vi "1.3.1-Serial Read.vi"(0 "Rx FPGA I/O":refnum<k21>="Rx", 1 "Read FIFO":refnum<k21>="Read FIFO", 7 "baud rate (9600)":u32=9600, 9 "data bits (8)":i32=8 min=5 max=8 step=1, 11 "parity (0:none)":enum16{"None", "Odd", "Even", "Mark", "Space"}(ring), 12 "stop bits (10: 1 bit)":u16(ring)=10 items=["1.0"=10, "1.5"=15, "2.0"=20], 13 "Invert Polarity?":bool) -> ()   [LabVIEW 2010]
uses:
  <vilib>/eio/EIONode/EIONode.xnode
  <vilib>/rvi/eio/nirviEIOImplementation/nirviEIOImplementation.xnode
  <vilib>/rvi/eio/common/nirviEmuClasses.ctl
  <vilib>/rvi/DataTransferAndStorage/Container/XNode/niFpgaContainer.xnode
  <vilib>/rvi/DataTransferAndStorage/Container/Common/niFpgaTransferTypeControl.ctl
  <vilib>/rvi/FIFO/Fifo_Types/niFpgaFifoControlLogicControl.ctl
  <vilib>/rvi/DataTransferAndStorage/Container/Common/niFpgaContainerMethod.ctl
  <vilib>/rvi/DataTransferAndStorage/Container/Common/niFpgaContainerMetaDataKey.ctl
  <vilib>/rvi/DataTransferAndStorage/FIFO/niFpgaPeerToPeerStreamState.ctl
  1.0-Hindbrain Global.vi
  <vilib>/rvi/eio/common/nirviEmuTemplateMethod_noerrors.vi
  Instance           1 27Saved   LV FPGA Serial Read .vi
  Instance           2 27Saved   LV FPGA Serial Read .vi
  <vilib>/rvi/DataTransferAndStorage/Container/Common/niFpgaContainerExecOnDevCompGetState.vi
  <vilib>/rvi/FIFO/Fifo_Resource/nirvififoEmulationSetSize.vi
  <vilib>/rvi/DataTransferAndStorage/Container/Common/niFpgaContainerGetUniqueNameForEmu.vi
  <vilib>/rvi/interface/RandomDataEmulation/nirviRandomDataFPGAFIFO.vi
  <vilib>/rvi/interface/RandomDataEmulation/niFpgaRandomDataHandleErrors.vi
  <vilib>/rvi/eio/common/nirviEmuReportErrorAndStop.vi
  Instance           3 27Saved   LV FPGA Serial Read .vi
  Instance           6 27Saved   LV FPGA Serial Read .vi
panel:
  out "Read: Transmission Error":bool
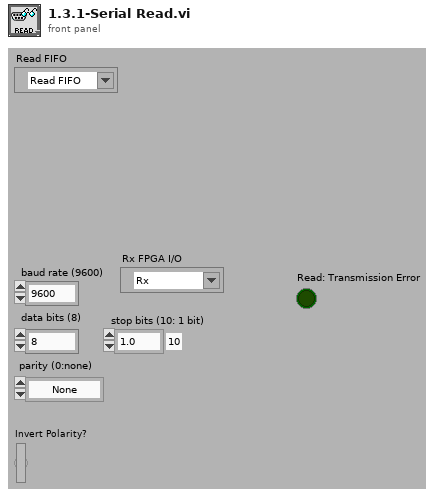
[diagram p1: front panel]
types:
  T1 = typedef "nirviEmuClasses.ctl" = enum16{"IO Read", "IO Write", "Method", "Property Read", "Property Write"}
  T2 = typedef "niFpgaFifoControlLogicControl.ctl" = enum16{"Slice Fabric", "Target Optimal", "Built-in"}
  T3 = typedef "niFpgaContainerMethod.ctl" = enum16{"<none>", "write", "read", "clear", "getNumberOfElementsToWrite", "getNumberOfElementsToRead", "enable", "disable", "flushAndDisable", "getStreamState", "readA", "readB", "dramWrite", "dramWriteWithByteEnables", "dramRequestData", "dramRetrieveData"}
  T4 = typedef "niFpgaTransferTypeControl.ctl" = enum16{"Target-Scoped", "Host to Target - DMA", "Target to Host - DMA", "Peer to Peer Reader", "Peer to Peer Writer", "Bidirectional"}
  T5 = typedef "niFpgaPeerToPeerStreamState.ctl" = enum16{"Unlinked", "Disabled", "Enabled", "Flushing"}
  T6 = typedef "niFpgaContainerMetaDataKey.ctl" = enum16{"FPGA FIFO", "FPGA Memory", "FPGA Register"}
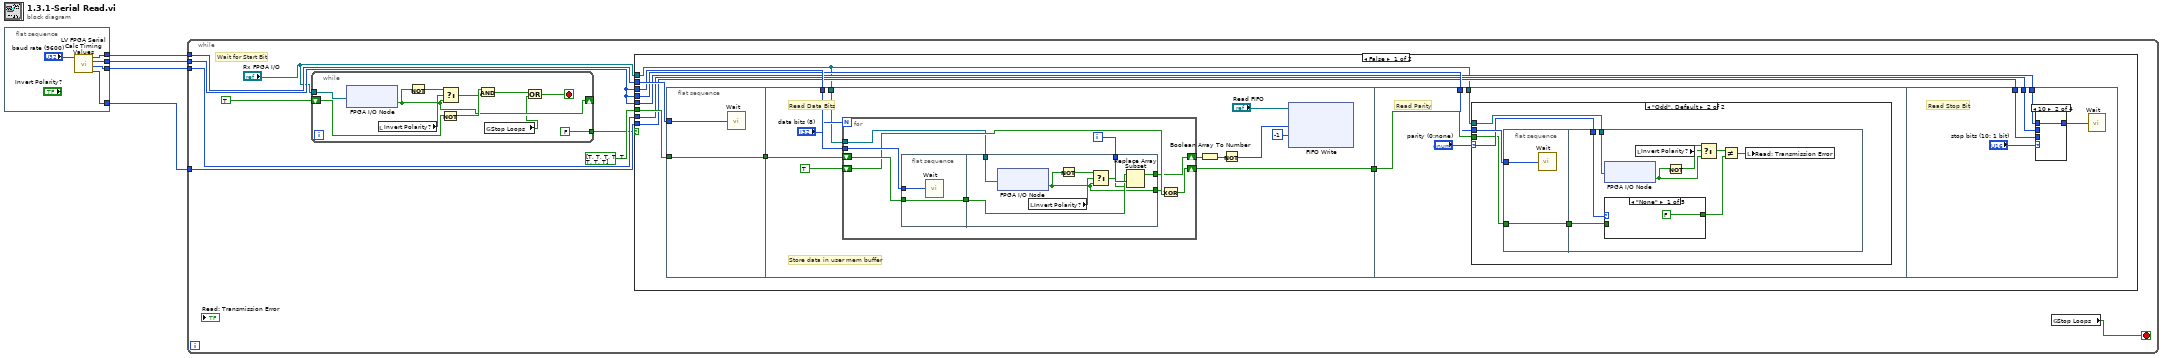
[diagram p0: block diagram]
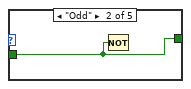
[diagram p3: hidden frame]
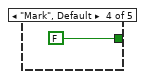
[diagram p5: hidden frame]
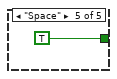
[diagram p6: hidden frame]
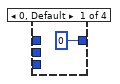
[diagram p7: hidden frame]
diagram:
  n1 = flat-sequence {
    tunnel: [w5] -> w3
    tunnel: [w8] -> w4
    tunnel: [w7] -> w2
    tunnel: [w6] -> w1
    frame #0 {
      n2 = call "LV FPGA Serial Calc Timing Values.vi"("baud rate (1000000)"="baud rate (9600)") -> ("Two Bit"=w6:u32, "One and Half Bit"=w7:u32, "One Bit"=w5:u32, "Half Bit"=w8:u32)  [unwired: 1 in, 2 out]
    }
  }
  n3 = while {
    tunnel: w1 -> [w17]
    tunnel: w2 -> [w16]
    tunnel: w3 -> [w15]
    tunnel: w4 -> [w14]
    stop <- w11 stop-if-true
    # "Wait for Start Bit"
    n4 = while {
      tunnel: [FALSE] -> w13
      shift-right: [w20] -> _
      shift-left: TRUE -> [w28]
      tunnel: "Rx FPGA I/O" -> [w24]
      stop <- w25 stop-if-true
      n5 = xnode "FPGA I/O Node"("FPGA I/O In"=w24) -> ("I/O Item"=w20:bool)  [unwired: 1 out]
      n6 = local read "Invert Polarity?"() -> (w22:bool)
      n7 = Not(x=w20) -> (.not. x?=w23:bool)
      n8 = Not(x=w28) -> (.not. x?=w27:bool)
      n9 = Select(t=w23, s=w22, f=w20) -> (s? t:f=w21:bool)
      n10 = And(x=w27, y=w21) -> (x .and. y?=w26:bool)
      n11 = global read "1.0-Hindbrain Global.vi" "Stop Loops"() -> (w19:bool)
      n12 = Or(x=w26, y=w19) -> (x .or. y?=w25:bool)
    }
    n13 = case shown="False" w13 {
      tunnel: bool[] [TRUE, TRUE, TRUE, TRUE, TRUE, TRUE, TRUE, TRUE] -> [w57 _]
      tunnel: w14 -> [w56 _]
      tunnel: w15 -> [w55 _]
      tunnel: w15 -> [w54 _]
      tunnel: w15 -> [w53 _]
      tunnel: w16 -> [w52 _]
      tunnel: w17 -> [w51 _]
      tunnel: "Rx FPGA I/O" -> [w49 _]
      frame False {
        n14 = flat-sequence {
          tunnel: [w60] -> w58
          tunnel: w57 -> [w60]
          tunnel: w56 -> [w59]
          tunnel: w58 -> [w71]
          tunnel: w55 -> [w70]
          tunnel: [w66] -> w50
          tunnel: w49 -> [w64]
          tunnel: w54 -> [w428]
          tunnel: w50 -> [w430]
          tunnel: w49 -> [w427]
          tunnel: w53 -> [w474]
          tunnel: w52 -> [w473]
          tunnel: w51 -> [w472]
          frame #0 {
            n15 = call "Wait"("Count(Ticks)"=w59) -> ()  [unwired: 1 out]
          }
          frame #1 {
            # "Store data in user mem buffer"
            # "Read Data Bits"
            n16 = for {
              N: "data bits (8)" -> [_]
              shift-right: [w391] -> w69
              shift-left: w71 -> [w397]
              tunnel: w70 -> [w395]
              shift-right: [w394] -> w66
              shift-left: TRUE -> [w393]
              tunnel: w64 -> [w389]
              i -> [w390]
              n17 = flat-sequence {
                tunnel: w397 -> [w399]
                tunnel: [w399] -> w396
                tunnel: w395 -> [w398]
                tunnel: w390 -> [w407]
                tunnel: w396 -> [w406]
                tunnel: [w405] -> w391
                tunnel: [w400] -> w392
                tunnel: w389 -> [w404]
                frame #0 {
                  n18 = call "Wait"("Count(Ticks)"=w398) -> ()  [unwired: 1 out]
                }
                frame #1 {
                  n19 = xnode "FPGA I/O Node"("FPGA I/O In"=w404) -> ("I/O Item"=w400:bool)  [unwired: 1 out]
                  n20 = local read "Invert Polarity?"() -> (w403:bool)
                  n21 = Not(x=w400) -> (.not. x?=w402:bool)
                  n22 = Select(t=w402, s=w403, f=w400) -> (s? t:f=w401:bool)
                  n23 = Replace Array Subset(array=w406, new element=w401, index=w407) -> (w405:bool[])
                }
              }
              n24 = Exclusive Or(1:w393, 2:w392) -> (0:w394:bool)
            }
            n25 = Boolean Array To Number(Boolean array=w69) -> (number=w68:u8)
            n26 = Not(x=w68) -> (.not. x?=w63:u8)
            n27 = xnode ("FIFO Write")("Element"=w63, "Timeout"=-1, "FIFO In"="Read FIFO") -> ()  [unwired: 2 out]
          }
          frame #2 {
            # "Read Parity"
            n28 = case shown="\"Odd\", Default" "parity (0:none)" {
              selector: "parity (0:none)" -> [_ w434]
              tunnel: w430 -> [_ w432]
              tunnel: w428 -> [_ w435]
              tunnel: w427 -> [_ w431]
              frame "None" {
              }
              frame "Odd", Default {
                n29 = flat-sequence {
                  tunnel: w435 -> [w437]
                  tunnel: [w436] -> w433
                  tunnel: w432 -> [w436]
                  tunnel: w434 -> [w446]
                  tunnel: w433 -> [w444]
                  tunnel: w431 -> [w442]
                  frame #0 {
                    n30 = call "Wait"("Count(Ticks)"=w437) -> ()  [unwired: 1 out]
                  }
                  frame #1 {
                    n31 = xnode "FPGA I/O Node"("FPGA I/O In"=w442) -> ("I/O Item"=w439:bool)  [unwired: 1 out]
                    n32 = case shown="\"None\"" w446 {
                      tunnel: w444 -> [_ w467 w468 _ _]
                      tunnel: [FALSE ("y") w467 w468 FALSE ("y") TRUE ("y")] -> w445
                      frame "None" {
                      }
                      frame "Odd" {
                        n33 = Not(x=w467) -> ()  [unwired: 1 out]
                      }
                      frame "Even" {
                      }
                      frame "Mark", Default {
                      }
                      frame "Space" {
                      }
                    }
                    n34 = local read "Invert Polarity?"() -> (w440:bool)
                    n35 = Not(x=w439) -> (.not. x?=w441:bool)
                    n36 = Select(t=w441, s=w440, f=w439) -> (s? t:f=w438:bool)
                    n37 = Not Equal?(x=w438, y=w445) -> (x != y?=w443:bool)
                    n38 = local write "Read: Transmission Error"(w443) -> ()
                  }
                }
              }
            }
          }
          frame #3 {
            # "Read Stop Bit"
            n39 = case shown="10" "stop bits (10: 1 bit)" {
              tunnel: w474 -> [_ w477 _ _]
              tunnel: w473 -> [_ _ w478 _]
              tunnel: w472 -> [_ _ _ w479]
              tunnel: [u32 0 ("One Bit") w477 w478 w479] -> w471
              frame 0, Default {
              }
              frame 10 {
              }
              frame 15 {
              }
              frame 20 {
              }
            }
            n40 = call "Wait"("Count(Ticks)"=w471) -> ()  [unwired: 1 out]
          }
        }
      }
      frame True {
      }
    }
    n41 = global read "1.0-Hindbrain Global.vi" "Stop Loops"() -> (w11:bool)
  }
